vi "Run.vi"(8 "error in (no error)":errorcluster, 11 "LUnit Test Case In":refnum<class "LUnit Inheriting Test Case.lvclass">) -> (0 "error out":errorcluster, 1 "Done?":bool, 2 "Results":T1[](array[typedef]), 3 "LUnit Test Case Out":refnum<class "LUnit Inheriting Test Case.lvclass">)   [LabVIEW 2020]
uses:
  LUnit Inheriting Test Case.lvclass
  Core/Result/Status.ctl
  Core/Result/Result.lvlib
  Core/Result/Type.ctl
  Core/Result/Result.ctl
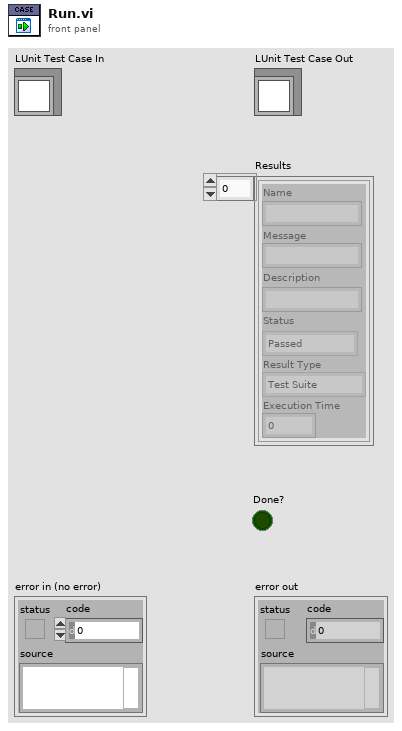
[diagram p1: front panel]
types:
  T1 = typedef "Result.lvlib/Result.ctl" = cluster{"Name":string, "Message":string, "Description":string, "Status":T2, "Result Type":T3, "Execution Time":dbl}
  T2 = typedef "Result.lvlib/Status.ctl" = enum16{"", "Passed", "Failed", "Error", "Skipped", "Setup Error", "Broken", "Teardown Error"}
  T3 = typedef "Result.lvlib/Type.ctl" = enum16{"Test Case", "Test Suite", "Test Run", "Pass", "Fail", "Skip", "Pass if", "Fail if", "Pass if Error", "Fail if Error", "Pass if Equal", "Fail if Equal"}
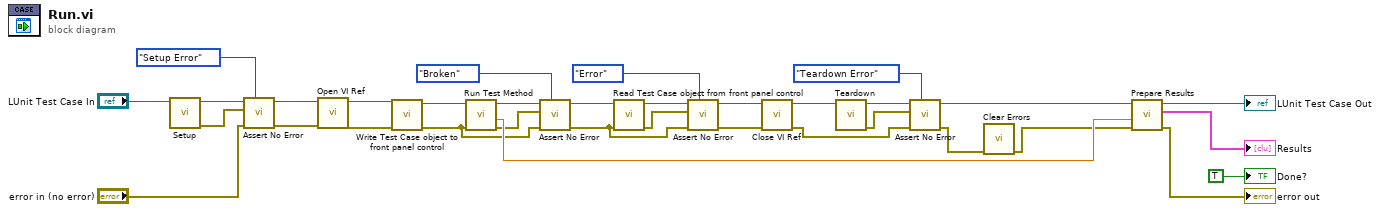
[diagram p0: block diagram]
diagram:
  n1 = call-dynamic "Setup.vi"("LUnit Test Case In"="LUnit Test Case In") -> ("error out"=w23:errorcluster, "LUnit Test Case Out"=w29:refnum<class "LUnit Inheriting Test Case.lvclass">)  [unwired: 9 in]
  n2 = call "Assert No Error.vi"("Status"=Status."Setup Error", "error In"="error in (no error)", "Assert error"=w23, "LUnit Test Case In"=w29) -> ("error out"=w30:errorcluster, "LUnit Test Case Out"=w28:refnum<class "LUnit Inheriting Test Case.lvclass">)  [unwired: 6 in]
  n3 = call "Open VI Ref.vi"("error in (no error)"=w30, "LUnit Test Case In"=w28) -> ("error out"=w22:errorcluster, "LUnit Test Case Out"=w21:refnum<class "LUnit Inheriting Test Case.lvclass">)  [unwired: 8 in]
  n4 = call "Write Test Case object to front panel control.vi"("error in (no error)"=w22, "LUnit Test Case In"=w21) -> ("error out"=w14:errorcluster, "LUnit Test Case Out"=w20:refnum<class "LUnit Inheriting Test Case.lvclass">)  [unwired: 8 in]
  n5 = call "Run Test Method.vi"("error in (no error)"=w14, "LUnit Test Case In"=w20) -> ("error out"=w15:errorcluster, "Execution Time"=w32:dbl, "LUnit Test Case Out"=w18:refnum<class "LUnit Inheriting Test Case.lvclass">)  [unwired: 7 in]
  n6 = call "Assert No Error.vi"("Status"=Status."Broken", "error In"=w14, "Assert error"=w15, "LUnit Test Case In"=w18) -> ("error out"=w9:errorcluster, "LUnit Test Case Out"=w17:refnum<class "LUnit Inheriting Test Case.lvclass">)  [unwired: 6 in]
  n7 = call "Read Test Case object from front panel control.vi"("error in (no error)"=w9, "LUnit Test Case In"=w17) -> ("error out"=w10:errorcluster, "LUnit Test Case Out"=w13:refnum<class "LUnit Inheriting Test Case.lvclass">)  [unwired: 8 in]
  n8 = call "Assert No Error.vi"("Status"=Status."Error", "error In"=w9, "Assert error"=w10, "LUnit Test Case In"=w13) -> ("error out"=w12:errorcluster, "LUnit Test Case Out"=w19:refnum<class "LUnit Inheriting Test Case.lvclass">)  [unwired: 6 in]
  n9 = call "Close VI Ref.vi"("error in (no error)"=w12, "LUnit Test Case In"=w19) -> ("error out"=w5:errorcluster, "LUnit Test Case Out"=w26:refnum<class "LUnit Inheriting Test Case.lvclass">)  [unwired: 8 in]
  n10 = call-dynamic "Teardown.vi"("LUnit Test Case In"=w26) -> ("error out"=w6:errorcluster, "LUnit Test Case Out"=w8:refnum<class "LUnit Inheriting Test Case.lvclass">)  [unwired: 9 in]
  n11 = call "Assert No Error.vi"("Status"=Status."Teardown Error", "error In"=w5, "Assert error"=w6, "LUnit Test Case In"=w8) -> ("error out"=w25:errorcluster, "LUnit Test Case Out"=w1:refnum<class "LUnit Inheriting Test Case.lvclass">)  [unwired: 6 in]
  n12 = call <vilib>:"Clear Errors.vi"("error in (no error)"=w25) -> ("error out"=w24:errorcluster)  [unwired: 5 in, 1 out]
  n13 = call "Prepare Results.vi"("error in (no error)"=w24, "Execution Time"=w32, "LUnit Test Case In"=w1) -> ("error out"=→"error out":errorcluster, "Results"=→"Results":T1[], "LUnit Test Case Out"=→"LUnit Test Case Out":refnum<class "LUnit Inheriting Test Case.lvclass">)  [unwired: 6 in]
  "Done?" <- TRUE ("Done?")
